vi "getOptCtrlTestSetting.vi"() -> (3 "Test Setting":T2)   [LabVIEW 2016]
doc: "Get the test setting of OptCtrl class."
uses:
  StrictDef/InstName.ctl
  OfcFunc.lvlib
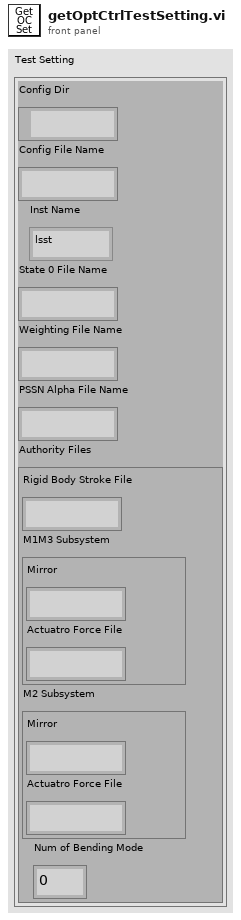
[diagram p1: front panel]
types:
  T1 = typedef "OfcFunc.lvlib/InstName.ctl" = enum16{"lsst", "comcam"}
  T2 = cluster{"Config Dir":path, "Config File Name":string, "Inst Name":T1, "State 0 File Name":string, "Weighting File Name":string, "PSSN Alpha File Name":string, "Authority Files":cluster{"Rigid Body Stroke File":string, "M1M3 Subsystem":cluster{"Mirror":string, "Actuatro Force File":string}, "M2 Subsystem":cluster{"Mirror":string, "Actuatro Force File":string}, "Num of Bending Mode":i32}}
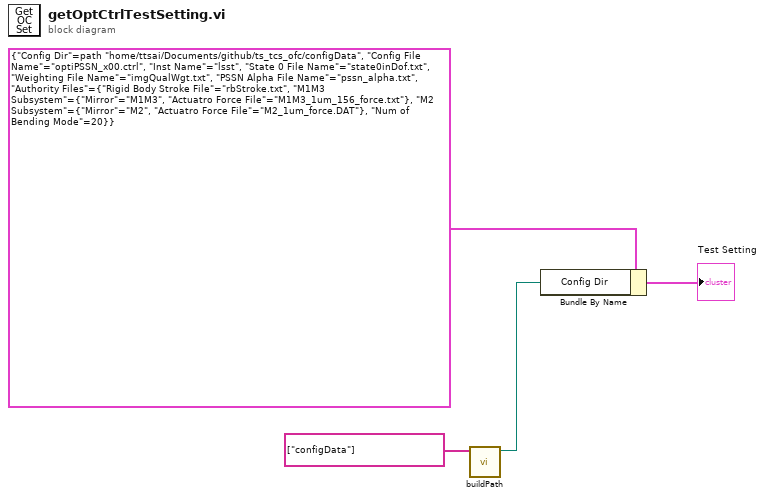
[diagram p0: block diagram]
diagram:
  n1 = call "buildPath.vi"("Path Name List"=string[] ["configData"]) -> ("New Path"=w2:path)  [unwired: 10 in]
  n2 = Bundle By Name(cluster=T2 {"Config Dir"=path "/home/ttsai/Documents/github/ts_tcs_ofc/configData", "Config File Name"="optiPSSN_x00.ctrl", "Inst Name"=enum."lsst", "State 0 File Name"="state0inDof.txt", "Weighting File Name"="imgQualWgt.txt", "PSSN Alpha File Name"="pssn_alpha.txt", "Authority Files"={"Rigid Body Stroke File"="rbStroke.txt", "M1M3 Subsystem"={"Mirror"="M1M3", "Actuatro Force File"="M1M3_1um_156_force.txt"}, "M2 Subsystem"={"Mirror"="M2", "Actuatro Force File"="M2_1um_force.DAT"}, "Num of Bending Mode"=20}} ("Configuration"), "Config Dir"=w2) -> (→"Test Setting":T2)
